vi "QuadratureEncoder.vi"() -> ()   [LabVIEW 2015]
doc: "DESCRIPTION:\nThis VI measures the rotation of a quadrature encoder. The quadrature encoder produces 96 pulses/revolution. \n\nNOTE: This VI only works with the BNC-2120 Connector Assembly.\n\n\n\nINSTRUCTIONS:\nEnter the appropriate device and counter number. Wire the BNC-2120 appropriately for the specified counter. By rotating the BNC quadrature encoder knob the vi will display the number of pulses and degrees rotated.\n\n\nKEY PARAMETERS:\n* device (Counter Group Config.vi): the device number you assigned to the E-Series DAQ device during configuration.\n* counter: (Counter Group Config.vi) the counter on the E-Series DAQ device you wish to use, either 0 or 1.\n\n\nI/O CONNECTIONS OVERVIEW:\nOn the BNC-2120, connect the CLK signal to the Source of the counter being used. \n For CTR0, connect CLK to CTR Source 0 (PFI8).\n For CTR1, connect CLK to CTR Source 1 (PFI3).\n\nConnect UP/DN signal to the direction line of the DAQ-STC as follows:\n For CTR0, connect UP/DN to DIO6.\n For CTR1, connect UP/DN to DIO7."
uses:
  <vilib>/myRIO/Common/Instrument Driver Framework/myRIO v1.0/Encoder/typedefs/Encoder Count Direction Enum.ctl
  <vilib>/myRIO/Express VI/Onboard IO/Encoder/Encoder Express VI.xnode
  <vilib>/myRIO/Instrument Drivers/Utilities/Utilities.lvlib
  <vilib>/myRIO/Instrument Drivers/Onboard IO/Encoder/vis/Read.vi
  <vilib>/myRIO/Instrument Drivers/Onboard IO/Encoder/Encoder.lvlib
  <vilib>/myRIO/Common/Instrument Driver Framework/myRIO v1.0/Encoder/typedefs/Encoder Signal Mode.ctl
  <vilib>/myRIO/Common/Instrument Driver Framework/myRIO v1.0/Encoder/typedefs/Encoder Channels Enum.ctl
  <vilib>/myRIO/Common/Instrument Driver Framework/Utilities/typedefs/Generic FPGA Reference.ctl
  <vilib>/myRIO/Common/Instrument Driver Framework/Utilities/typedefs/myRIO v1.0 Reference.ctl
  <vilib>/myRIO/Common/Instrument Driver Framework/Utilities/typedefs/Hardware Version Enum.ctl
  <vilib>/myRIO/Common/Instrument Driver Framework/Utilities/typedefs/myRIO Generic Hardware Reference.ctl
  <vilib>/myRIO/Instrument Drivers/Onboard IO/Encoder/typedefs/Encoder Reference.ctl
  <vilib>/myRIO/Instrument Drivers/Onboard IO/Encoder/vis/myRIO Encoder Open.xnode
  <vilib>/myRIO/Common/Instrument Driver Framework/Utilities/vis/Is FPGA Ref Available.vi
  <vilib>/myRIO/Common/Instrument Driver Framework/myRIO v1.0/Encoder/vis/myRIO v1.1 Open Encoder.vi
  <vilib>/myRIO/Common/Instrument Driver Framework/myRIO v1.0/Encoder/vis/myRIO v1.0 Configure Encoder.vi
  <vilib>/myRIO/Common/Instrument Driver Framework/myRIO v1.0/Encoder/typedefs/Encoder Configuration v1.0.ctl
  <vilib>/userdefined/High Color/nirio_resource_hc.ctl
panel:
  out "Degrees":dbl(knob) scale=0.0..360.0 scale format="%#.1f"
  out "Number of Revolutions":dbl
  out "Total Degrees Rotated":dbl format="%.2f"
  out "CLK pulses":i32 caption="CLK pulses 2"
  in  "stop":bool
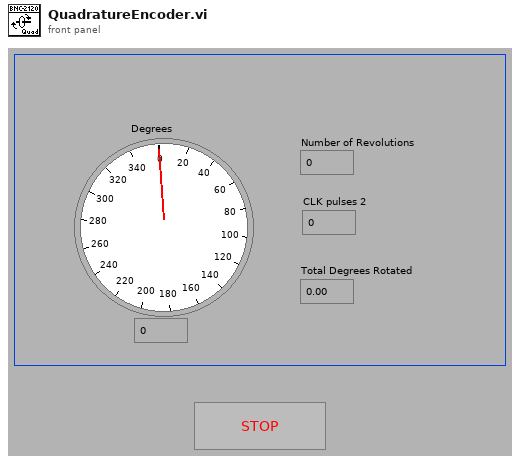
[diagram p1: front panel]
types:
  T1 = typedef "Encoder.lvlib/Encoder Reference.ctl" = cluster{"myRIO Reference":T2, "Encoder Channels Enum":T6}
  T2 = typedef "myRIO Generic Hardware Reference.ctl" = cluster{"myRIO Model":T3, "myRIO Hardware Reference":T4}
  T3 = typedef "Hardware Version Enum.ctl" = enum16{"Unknown", "myRIO-1900", "myRIO-1950", "roboRIO"}
  T4 = typedef "myRIO v1.0 Reference.ctl" = cluster{"Generic FPGA Reference":T5, "Allow multiple opens":bool}
  T5 = typedef "Generic FPGA Reference.ctl" = refnum<k20>
  T6 = typedef "Encoder Channels Enum.ctl" = enum16{"Not Connected", "C/ENC0", "C/ENC1", "A/ENC", "B/ENC", "DIO/ENC0", "DIO/ENC1", "DIO/ENC2", "DIO/ENC3", "DIO/ENC4"}
  T7 = typedef "Encoder Signal Mode.ctl" = enum16{"Quadrature phase signal", "Step and direction signal"}
  T8 = typedef "nirio_resource_hc.ctl" = tag
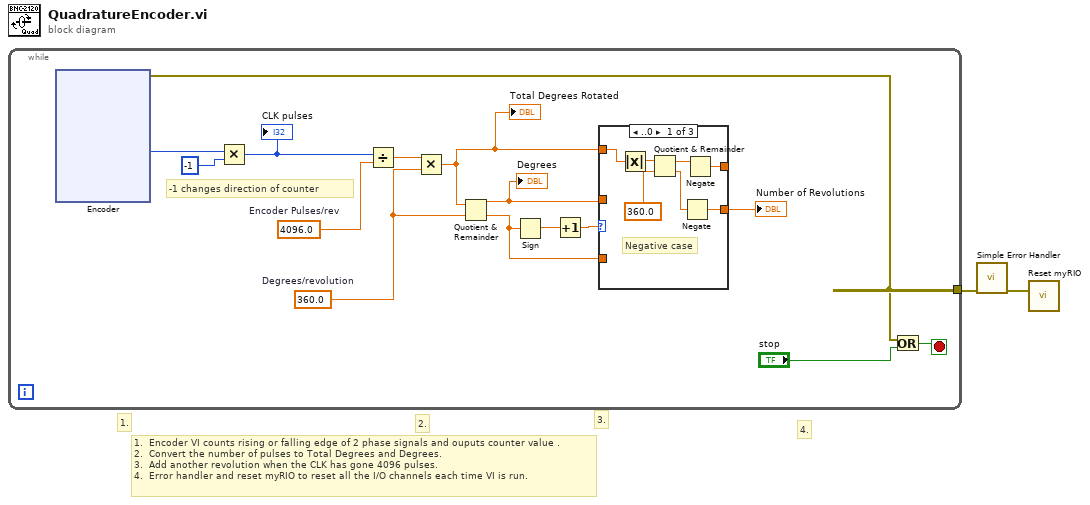
[diagram p0: block diagram]
diagram:
  # "4."
  # "3."
  # "2."
  # "1."
  # "1.  Encoder VI counts rising or falling edge of 2 phase signals and ouputs counter value .\n2.  Convert the number of pulses to Total Degrees and Degrees.\n3.  Add another revolution when the CLK has gone 4096 pulses.\n4.  Error handler and reset myRIO to reset all the I/O channels each time VI is run."
  n1 = while {
    tunnel: [w10] -> w1
    stop <- w16 stop-if-true
    w7 = 4096.0  # Encoder Pulses/rev
    w4 = 360.0  # Degrees/revolution
    # "-1 changes direction of counter"
    n2 = xnode "Encoder"() -> ("Counter Value"=w8:i32, "error out"=w10:errorcluster)  [unwired: 2 in, 2 out]
    n3 = Multiply(x=w8, y=-1) -> (x*y=w6:i32)
    "CLK pulses" <- w6
    n4 = Divide(x=w6, y=w7) -> (x/y=w5:dbl)
    n5 = Multiply(x=w5, y=w4) -> (x*y=w3:dbl)
    "Total Degrees Rotated" <- w3
    n6 = Quotient & Remainder(x=w3, y=w4) -> (x-y*floor(x/y)=w11:dbl, floor(x/y)=w12:dbl)
    "Degrees" <- w11
    n7 = Sign(1:w12) -> (0:w15:dbl)
    n8 = Increment(x=w15) -> (x+1=w14:dbl)
    n9 = case shown="..0" w14 {
      tunnel: w3 -> [w70 _ _]
      tunnel: w11 -> [_ w72 w74]
      tunnel: [w65 w71 w73] -> w13
      tunnel: [w64 w72 w74] -> _
      tunnel: w12 -> [_ w71 w73]
      frame ..0 {
        # "Negative case"
        n10 = Absolute Value(x=w70) -> (abs(x)=w69:dbl)
        n11 = Quotient & Remainder(x=w69, y=360.0) -> (x-y*floor(x/y)=w68:dbl, floor(x/y)=w66:dbl)
        n12 = Negate(x=w66) -> (-x=w65:dbl)
        n13 = Negate(x=w68) -> (-x=w64:dbl)
      }
      frame 1 {
      }
      frame 2.. {
      }
    }
    "Number of Revolutions" <- w13
    n14 = Or(x=w10, y="stop") -> (x .or. y?=w16:bool)
  }
  n15 = call <vilib>:"Simple Error Handler.vi"("error in (no error)"=w1) -> ("error out"=w2:errorcluster)  [unwired: 4 in, 4 out]
  n16 = call <vilib>:"Reset myRIO.vi"("error in (no error)"=w2) -> ()  [unwired: 10 in, 1 out]
